vi "Generate Packages List.vi"(8 "error in (no error)":errorcluster, 10 "Repos":refnum<class "Repo.lvclass">[](array[class]), 11 "LabVIEW Web Service":refnum<class "Web Service.lvclass">) -> (0 "error out":errorcluster, 3 "LabVIEW Web Service out":refnum<class "Web Service.lvclass">)   [LabVIEW 2016, in "Packages.lvlib"]
uses:
  Packages.lvlib
  Repo_class/Repo.lvclass
  <vilib>/wsapi/Web Service.lvclass
  Repo_class/Repo.lvclass/Repo.ctl
  Package_class/Package.lvclass/Package.ctl
  Package Version_class/Package Version.lvclass/Package Version.ctl
  Repo_class/Read Packages.vi
  Package_class/Read DisplayName.vi
  Package_class/Read Versions.vi
  Package_class/Read Name.vi
  Package Version_class/Read Vendor.vi
  Package_class/Package.lvclass
  Package Version_class/Package Version.lvclass
  WSsupport/WSsupport.lvlib
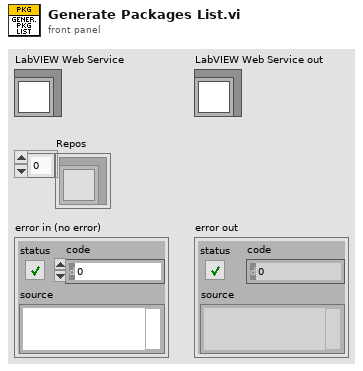
[diagram p1: front panel]
types:
  T1 = enum16{"open", "replace", "create", "open or create", "replace or create", "replace or create with confirmation"}
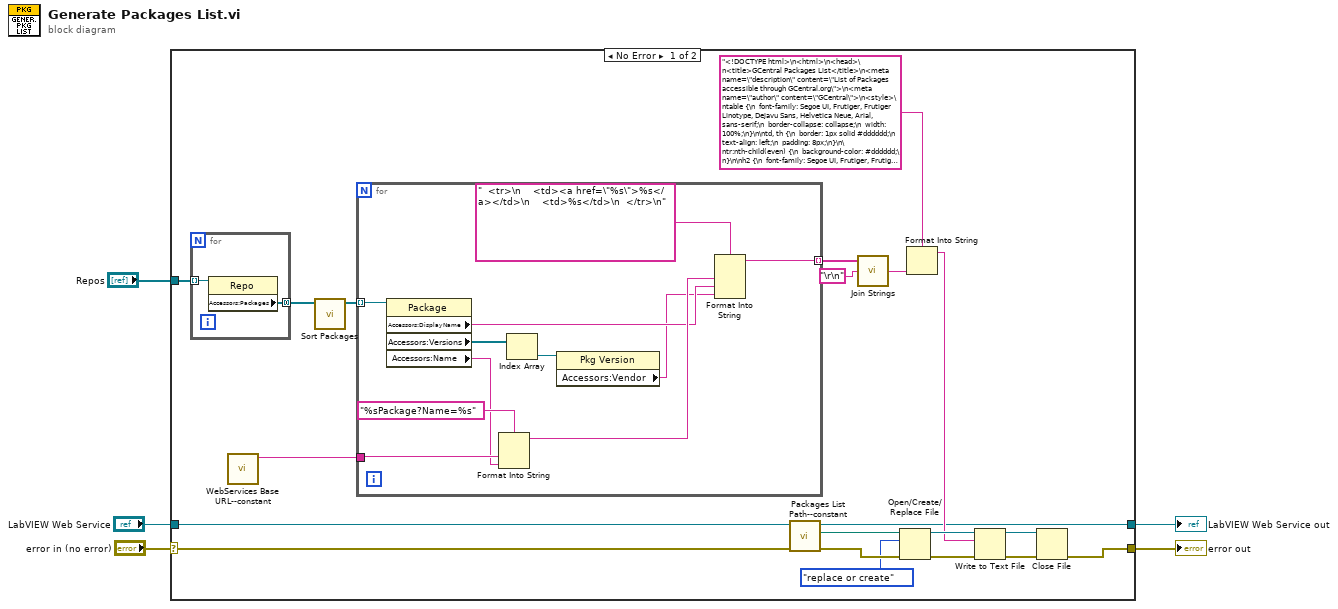
[diagram p0: block diagram]
diagram:
  n1 = case shown="No Error" "error in (no error)" {
    selector: "error in (no error)" -> [w21 w40]
    tunnel: "Repos" -> [w25 _]
    tunnel: [w11 w40] -> w3
    tunnel: "LabVIEW Web Service" -> [w7 w39]
    tunnel: [w6 w39] -> w1
    frame No Error {
      n2 = for {
        tunnel: [w38] -> w24 mode=concatenating
        tunnel: w25 -> [w37] mode=indexing
        n3 = property class="Repo"(reference=w37) -> ("Accessors:Packages"=w38:refnum<class "Package.lvclass">[])  [unwired: 1 in, 2 out]
      }
      n4 = call "WebServices Base URL--constant.vi"() -> ("WebServices Base URL"=w22:string)  [unwired: 11 in]
      n5 = call "Sort Packages.vi"("Packages"=w24) -> ("Sorted Packages"=w23:refnum<class "Package.lvclass">[])  [unwired: 10 in]
      n6 = for {
        tunnel: w23 -> [w36] mode=indexing
        tunnel: w22 -> [w35]
        tunnel: [w26] -> w20 mode=indexing
        n7 = property class="Package"(reference=w36) -> ("Accessors:DisplayName"=w29:string, "Accessors:Versions"=w32:refnum<class "Package Version.lvclass">[], "Accessors:Name"=w33:string)  [unwired: 1 in, 2 out]
        n8 = Format Into String(format string="%sPackage?Name=%s", w35, w33) -> (resulting string=w30:string)  [unwired: 2 in, 1 out]
        n9 = Index Array(array=w32) -> (element=w31:refnum<class "Package Version.lvclass">)  [unwired: 1 in]
        n10 = property class="Pkg Version"(reference=w31) -> ("Accessors:Vendor"=w28:string)  [unwired: 1 in, 2 out]
        n11 = Format Into String(format string="  <tr>\n    <td><a href=\"%s\">%s</a></td>\n    <td>%s</td>\n  </tr>\n", w30, w29, w28) -> (resulting string=w26:string)  [unwired: 2 in, 1 out]
      }
      n12 = call "Packages List Path--constant.vi"("error in (no error)"=w21, "LabVIEW Web Service"=w7) -> ("error out"=w16:errorcluster, "Packages index path"=w14:path, "LabVIEW Web Service out"=w6:refnum<class "Web Service.lvclass">)  [unwired: 7 in]
      n13 = call <vilib>:"Join Strings.vi"("Separator (,)"="\r\n", "Strings In"=w20) -> ("String"=w18:string)  [unwired: 1 in]
      n14 = Open/Create/Replace File(file path (use dialog)=w14, error in=w16, operation (0:open)=T1."replace or create") -> (refnum out=w10:refnum<file>, error out=w15:errorcluster)  [unwired: 3 in, 1 out]
      n15 = Format Into String(format string="<!DOCTYPE html>\n<html>\n<head>\n<title>GCentral Packages List</title>\n<meta name=\"description\" content=\"List of Packages accessible through GCentral.org\">\n<meta name=\"author\" content=\"GCentral\">\n<style>\ntable {\n  font-family: Segoe UI, Frutiger, Frutiger Linotype, Dejavu Sans, Helvetica Neue, Arial, sans-serif;\n  border-collapse: collapse;\n  width: 100%;\n}\n\ntd, th {\n  border: 1px solid #dddddd;\n  text-align: left;\n  padding: 8px;\n}\n\ntr:nth-child(even) {\n  background-color: #dddddd;\n}\n\nh2 {\n  font-family: Segoe UI, Frutiger, Frutiger Linotype, Dejavu Sans, Helvetica Neue, Arial, sans-serif;\n  text-align:center;\n}\n\n.center {\n  display: block;\n  margin-left: auto;\n  margin-right: auto;\n  width: 50%;\n}\n</style>\n</head>\n<body>\n\n<picture>\n  <img src=\"https://demo.studiobods.com/GCentral_Indexer/images/logo.png\" alt=\"Logo\" style=\"width:auto;\" class=\"center\">\n</picture>\n\n<h2>GCentral Packages List</h2>\n\n<table align=\"center\">\n  <tr>\n    <th>Package</th>\n    <th>Vendor</th>\n  </tr>%s\n</table>\n\n</body>\n</html>\n", w18) -> (resulting string=w8:string)  [unwired: 2 in, 1 out]
      n16 = Write to Text File(file (use dialog)=w10, text=w8, error in=w15) -> (refnum out=w9:refnum<file>, error out=w12:errorcluster)  [unwired: 1 in, 1 out]
      n17 = Close File(refnum=w9, error in=w12) -> (error out=w11:errorcluster)  [unwired: 1 out]
    }
    frame Error {
    }
  }
  "error out" <- w3
  "LabVIEW Web Service out" <- w1
